vi "calculateWaveformTime.vi"(8 "error in (no error)":errorcluster, 11 "PeriodicWave in":refnum<class "PeriodicWave.lvclass">) -> (0 "error out":errorcluster, 2 "Waveform Time":dbl[unit], 3 "PeriodicWave out":refnum<class "PeriodicWave.lvclass">)   [LabVIEW 2015, in "PeriodicWave.lvclass"]
uses:
  PeriodicWave.lvclass
  PeriodicWave.lvclass/PeriodicWave.ctl
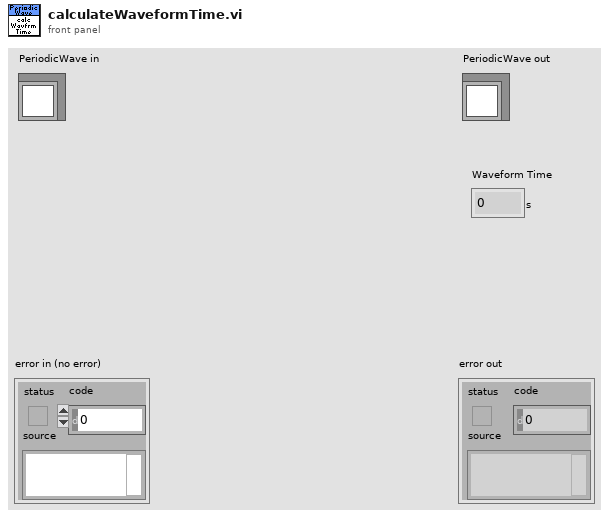
[diagram p1: front panel]
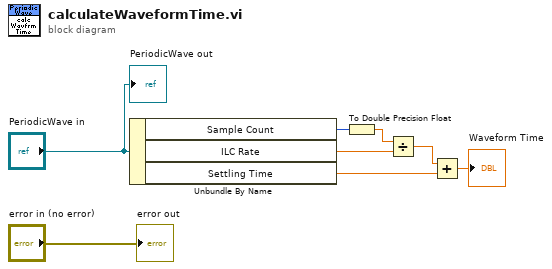
[diagram p0: block diagram]
diagram:
  n1 = Unbundle By Name("PeriodicWave in") -> ("Sample Count"=w5:u32, "ILC Rate"=w4:dbl[unit], "Settling Time"=w2:dbl[unit])
  n2 = To Double Precision Float(number=w5) -> (double precision float=w6:dbl)
  n3 = Divide(x=w6, y=w4) -> (x/y=w3:dbl[unit])
  n4 = Add(x=w3, y=w2) -> (x+y=→"Waveform Time":dbl[unit])
  "error out" <- "error in (no error)"
  "PeriodicWave out" <- "PeriodicWave in"
